vi "IdentityCheck.vi"(8 "error in (no error)":errorcluster, 11 "DeviceInterface in":refnum<class "DeviceInterface.lvclass">) -> (0 "error out":errorcluster, 3 "DeviceInterface out":refnum<class "DeviceInterface.lvclass">)   [LabVIEW 2013, in "DeviceInterface.lvclass"]
doc: "An das Gerät wird eine Nachricht geschickt, in der Regel der Befehl idn?. Anhand der Antwort kann erkannt werden ob das erwartete Gerät angeschlossen ist."
uses:
  DeviceInterface.lvclass
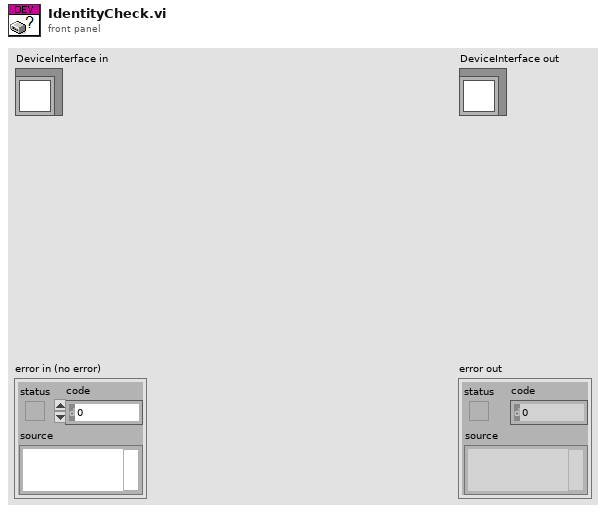
[diagram p1: front panel]
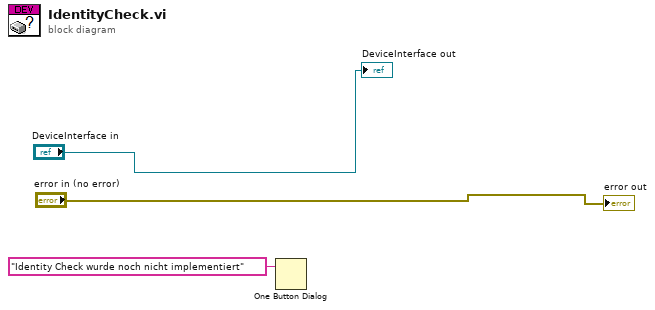
[diagram p0: block diagram]
diagram:
  n1 = One Button Dialog(message="Identity Check wurde noch nicht implementiert" ("Nachricht")) -> ()  [unwired: 1 in, 1 out]
  "error out" <- "error in (no error)"
  "DeviceInterface out" <- "DeviceInterface in"
